vi "ATR.vi"() -> ()   [LabVIEW 2017]
panel:
  out "deleted portion 3":string[](array[string])
  out "ArrEbay 2":string[][](array[string])
  out "output array":string[][](array[string])
  out "ATR 2":string[][](table)=[["Test Communication", "-", "-", "-", "-", ""], ["Set S/N", "-", "-", "-", "-", ""], ["Set Board Number", "-", "-", "-", "-", ""], [" ", "", "", "", "", ""], ["Test Communication", "-", "-", "-", "-", ""], ["Get S/N", "-", "-", "-", "", ""], ["Get Board Number", "-", "-", "-", "", ""], ["Get FW", "-", "-", "-", "", ""], ["Enable Motor", "", "", "", "", ""], ["Small position command", "", "", "", "", ""], ["Measure delta", "", "", "", "", ""], ["Velocity command", "", "", "", "", ""]] caption="ATR"
  out "ATR":string[][](table)=[["Test Communication", "-", "-", "-", "-", ""], ["Set S/N", "-", "-", "-", "-", ""], ["Set Board Number", "-", "-", "-", "-", ""], [" ", "", "", "", "", ""], ["Test Communication", "-", "-", "-", "-", ""], ["Get S/N", "-", "-", "-", "", ""], ["Get Board Number", "-", "-", "-", "", ""], ["Get FW", "-", "-", "-", "", ""], ["Enable Motor", "", "", "", "", ""], ["Small position command", "", "", "", "", ""], ["Measure delta", "", "", "", "", ""], ["Velocity command", "", "", "", "", ""]]
  out "Array 2":string[](array[string])
  out "Array":string[](array[string])
  out "deleted portion 2":string[](array[string])
  out "deleted portion":string[](array[string])
  out "ArrAHU":string[][](array[string])
  out "ArrEbay":string[][](array[string])
  out "Mort Temp":string[][](array[string])
  out "Aux":string[][](array[string])
  out "Burnin":string[][](array[string])
  out "Temp Algo":string[][](array[string])
  out "Speed":string[][](array[string])
  out "Tempreature calibration":string[][](array[string])
  out "StopTime":string[][](array[string])
  out "Enable":string[][](array[string])
  out "Communication":string[][](array[string])
  out "Visual Inspection":string[][](array[string])
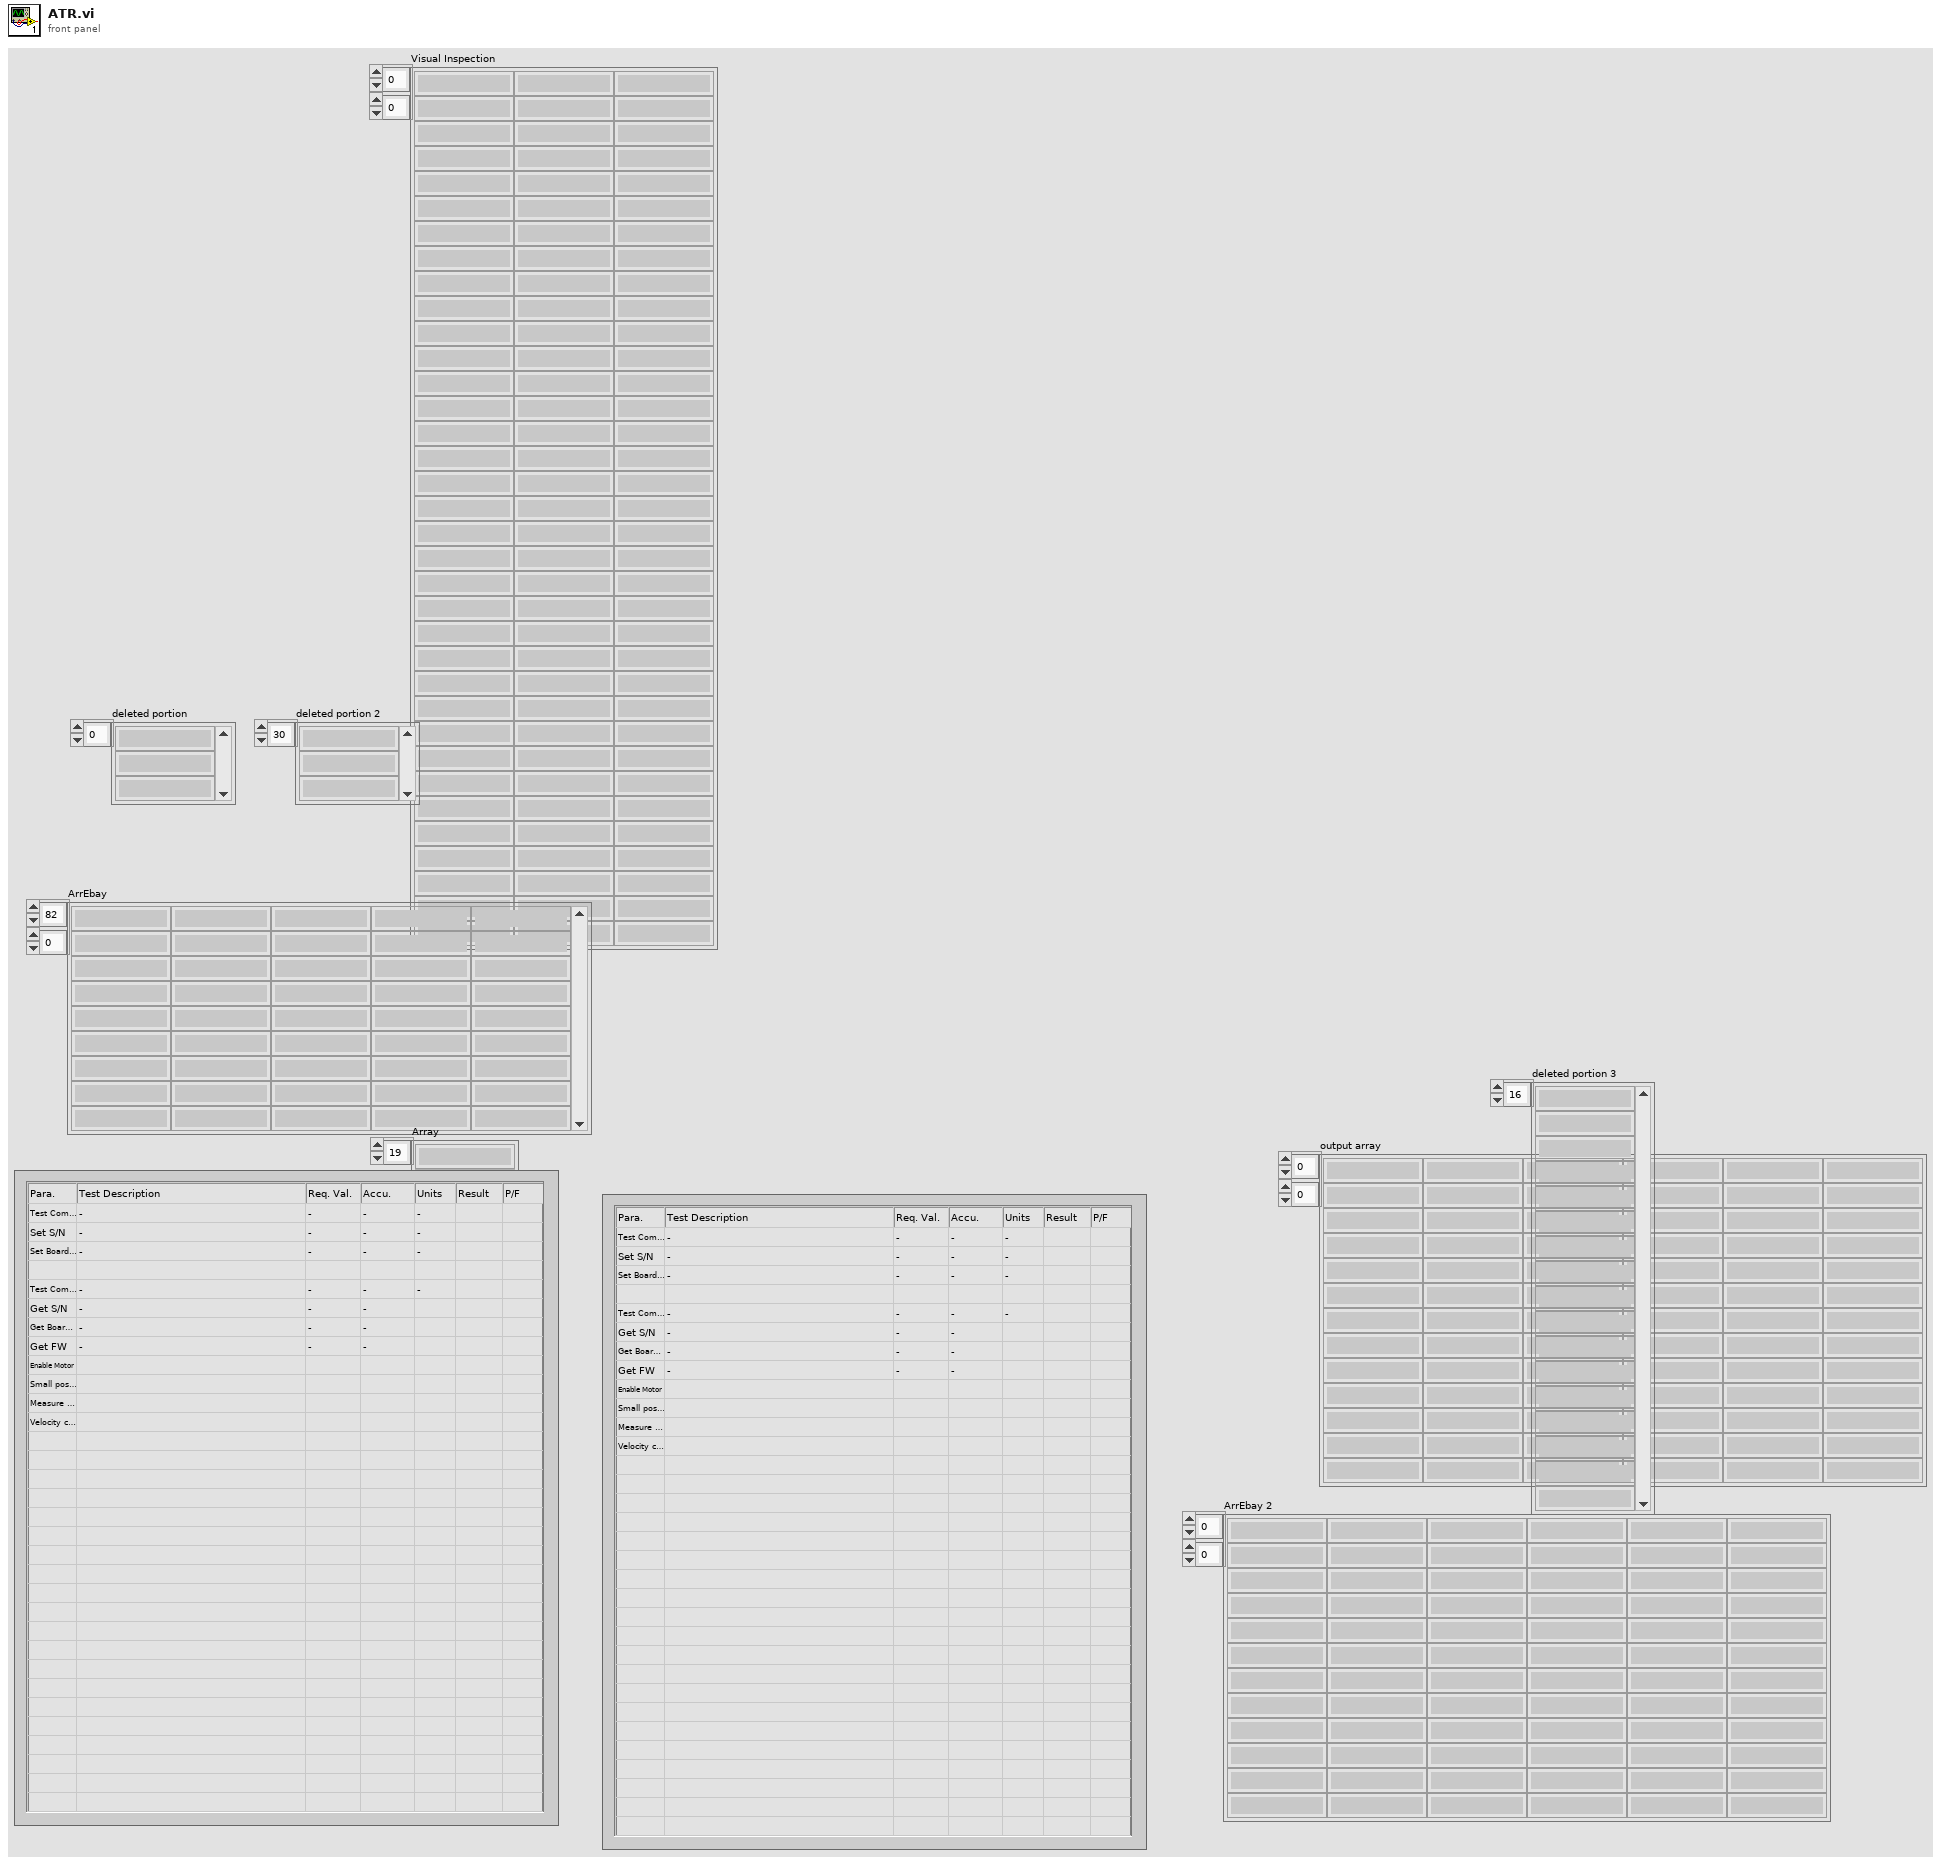
[diagram p1: front panel]
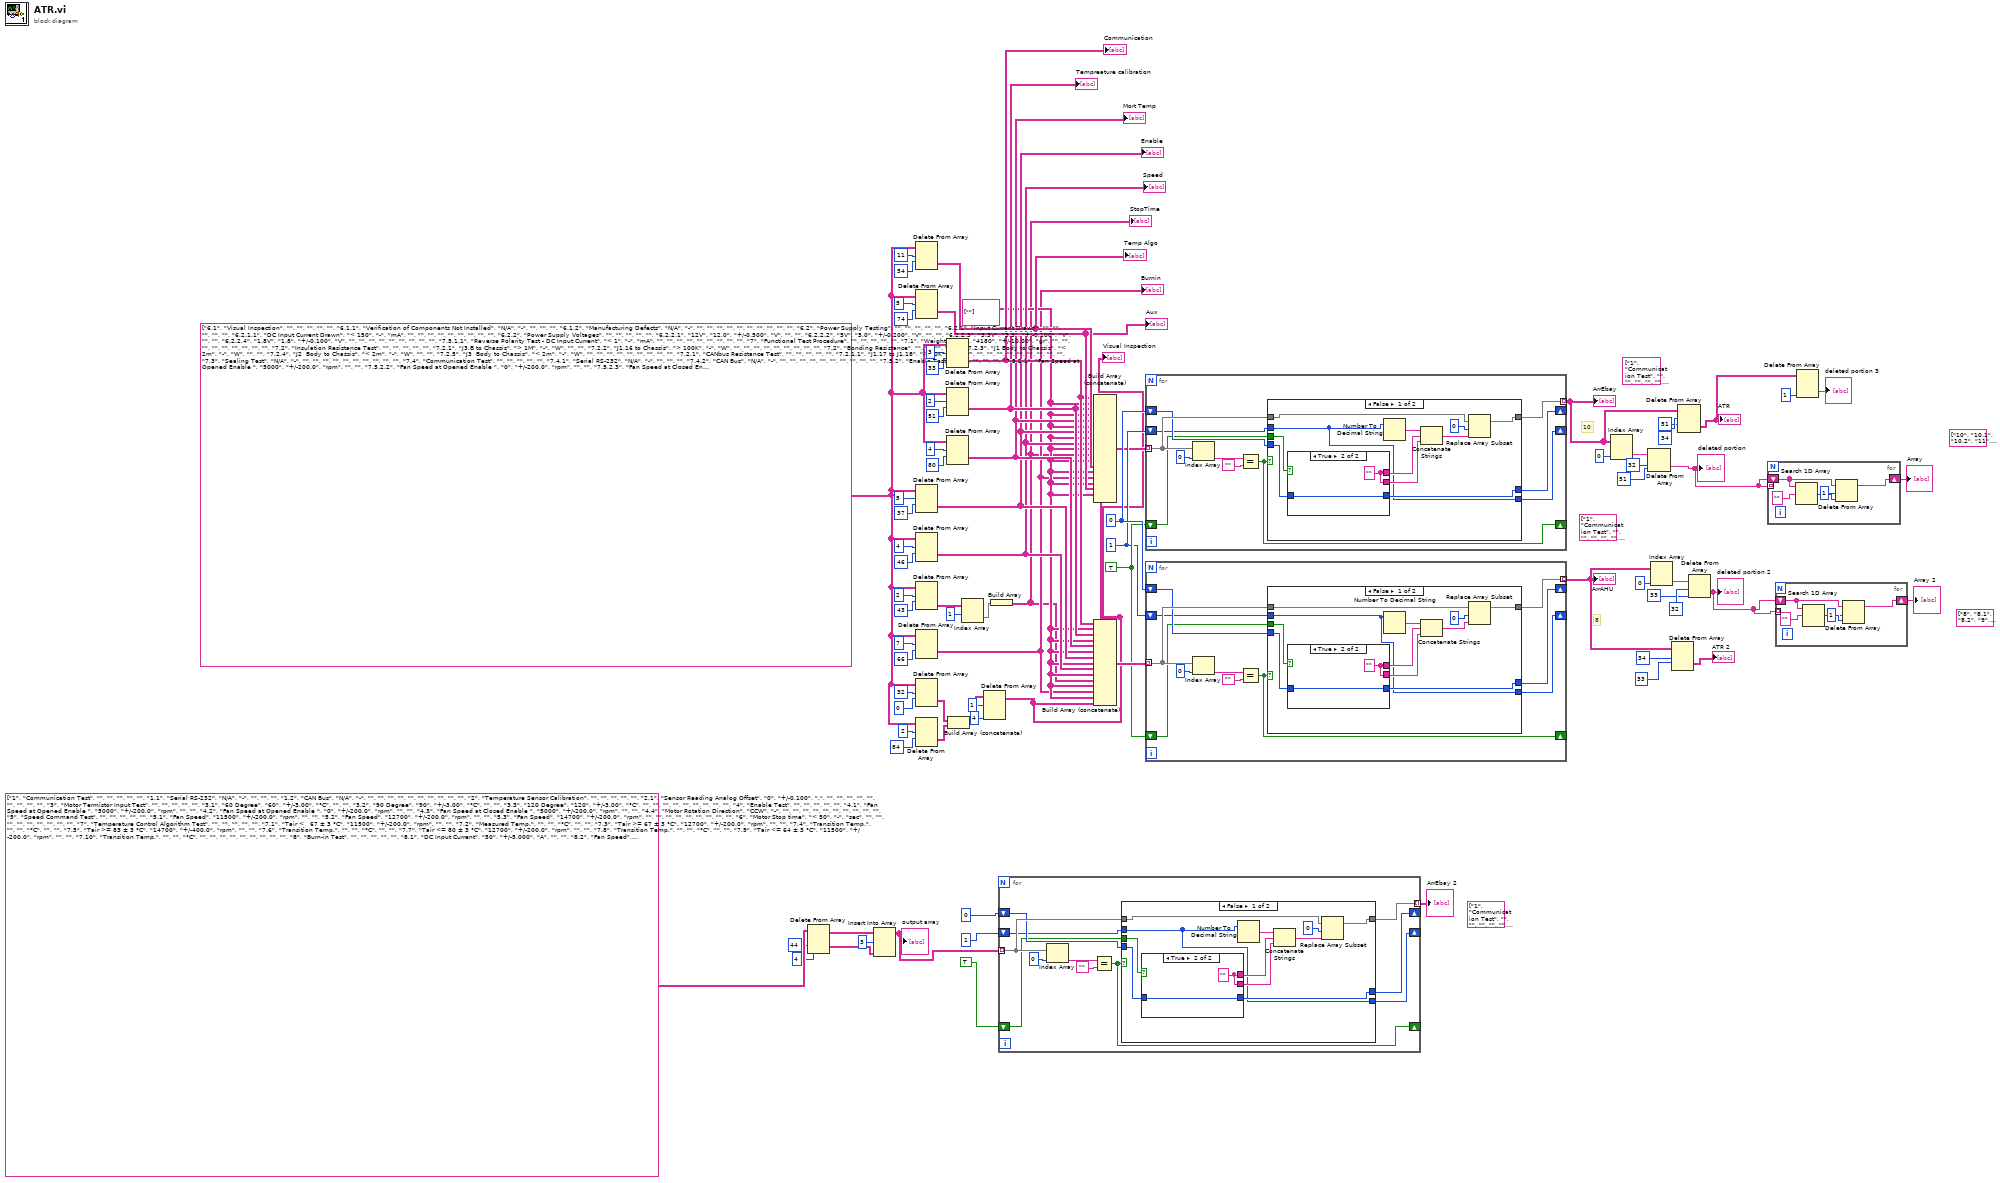
[diagram p0: block diagram]
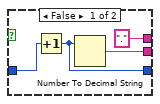
[diagram p2: hidden frame]
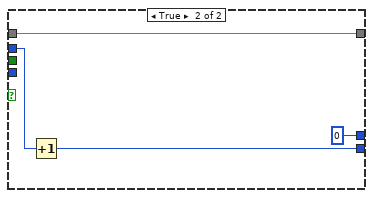
[diagram p3: hidden frame]
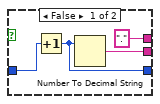
[diagram p4: hidden frame]
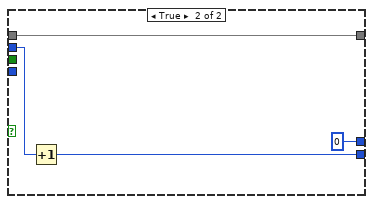
[diagram p5: hidden frame]
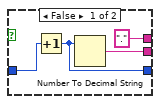
[diagram p6: hidden frame]
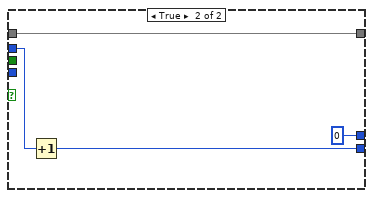
[diagram p7: hidden frame]
diagram:
  (unwired) string[][] [["1", "Communication Test", "", "", "", "", ""], ["1.1", "Serial RS-232", "N/A", "-", "", "", ""], ["1.2", "CAN Bus", "N/A", "-", "", "", ""], ["", "", "", "", "", "", ""], ["2", "Auxiliary Fan Test", "", "", "", "", ""], ["2.1", "Fan status-ON", "ON", "-", "-", "", ""], ["2.2", "Fan status-OFF", "OFF", "-", "-", "", ""], ["", "", "", "", "", "", ""], ["3", "Temperature Sensor Calibration", "", "", "", "", ""], ["3.1", "Sensor Reading Analog Offset", "0", "+/-0.100", ".", "", ""], ["", "", "", "", "", "", ""], ["4", "Motor Termistor Input Test", "", "", "", "", ""], ["4.1", "60 Degree", "60", "+/-3.00", "°C", "", ""], ["4.2", "90 Degree", "90", "+/-3.00", "°C", "", ""], ["4.3", "120 Degree", "120", "+/-3.00", "°C", "", ""], ["", "", "", "", "", "", ""], ["5", "Enable Test", "", "", "", "", ""], ["5.1", "Fan Speed at Opened Enable ", "5000", "+/-200.0", "rpm", "", ""], ["5.2", "Fan Speed at Opened Enable ", "0", "+/-200.0", "rpm", "", ""], ["5.3", "Fan Speed at Closed Enable ", "5000", "+/-200.0", "rpm", "", ""], ["5.4", "Motor Rotation Direction", "CCW", "-", "", "", ""], ["", "", "", "", "", "", ""], ["6", "Speed Command Test", "", "", "", "", ""], ["6.1", "Fan Speed", "11500", "+/-200.0", "rpm", "", ""], ["6.2", "Fan Speed", "12700", "+/-200.0", "rpm", "", ""], ["6.3", "Fan Speed", "14700", "+/-200.0", "rpm", "", ""], ["", "", "", "", "", "", ""], ["7", "Motor Stop time", "< 50", "-", "sec", "", ""], ["", "", "", "", "", "", ""], ["8", "Temperature Control Algorithm Test", "", "", "", "", ""], ["8.1", "Tair <   67 ± 3 °C", "11500", "+/-200.0", "rpm", "", ""], ["8.2", "Measured Temp.", "", "", "°C", "", ""], ["8.3", "Tair >= 67 ± 3 °C", "12700", "+/-200.0", "rpm", "", ""], ["8.4", "Transition Temp.", "", "", "°C", "", ""], ["8.5", "Tair >= 83 ± 3 °C", "14700", "+/-400.0", "rpm", "", ""], ["8.6", "Transition Temp.", "", "", "°C", "", ""], ["8.7", "Tair <= 80 ± 3 °C", "12700", "+/-200.0", "rpm", "", ""], ["8.8", "Transition Temp.", "", "", "°C", "", ""], ["8.9", "Tair <= 64 ± 3 °C", "11500", "+/-200.0", "rpm", "", ""], ["8.10", "Transition Temp.", "", "", "°C", "", ""], ["", "", "", "", "", "", ""], ["9", "Burn-in Test", "", "", "", "", ""], ["9.1", "DC Input Current", "50", "+/-5.000", "A", "", ""], ["9.2", "Fan Speed", "14700", "+/-200.0", "rpm", "", ""], ["9.3", "Ambient Temperature", "25", "+/-13.00", "°C", "", ""], ["9.4", "After 10 min of operation", "", "-", "°C", "", ""], ["9.5", "After 20 min of operation", "", "-", "°C", "", ""], ["9.6", "After 30 min of operation", "", "-", "°C", "", ""], ["", "", "", "", "", "", ""], ["10", "Visual Inspection", "", "", "", "", ""], ["10.1", "Verification of Components Not Installed", "N/A", "-", "", "", ""], ["10.2", "Manufacturing Defects", "N/A", "-", "", "", ""], ["", "", "", "", "", "", ""], ["11", "Power Supply Testing", "", "", "", "", ""], ["11.1", "DC Input Current Drawn", "150", "+/-10.00", "mA", "", ""], ["", "", "", "", "", "", ""], ["12", "Power Supply Voltages", "", "", "", "", ""], ["12.1", "12V", "12.0", "+/-0.500", "V", "", ""], ["12.2", "5V", "5.0", "+/-0.200", "V", "", ""], ["12.3", "3.3V", "3.3", "+/-0.100", "V", "", ""], ["12.4", "1.8V", "1.8", "+/-0.100", "V", "", ""], ["", "", "", "", "", "", ""], ["13", "Reverse Polarity Test - DC Input Current", "< 1", "-", "mA", "", ""], ["", "", "", "", "", "", ""], ["14", "Functional Test Procedure", "", "", "", "", ""], ["14.1", "Weight Check", "4180", "+/-100.0", "gr", "", ""], ["", "", "", "", "", "", ""], ["15", "Insulation Resistance Test", "", "", "", "", ""], ["15.1", "J3.B to Chassis", "> 1M", "-", "ohms", "", ""], ["15.2", "J1.16 to Chassis", "> 100K", "-", "ohms", "", ""], ["", "", "", "", "", "", ""], ["16", "Bonding Resistance", "", "", "", "", ""], ["16.1", "J1 Body to Chassis", "< 2m", "-", "ohms", "", ""], ["16.2", "J2  Body to Chassis", "< 2m", "-", "ohms", "", ""], ["16.3", "J3  Body to Chassis", "< 2m", "-", "ohms", "", ""], ["", "", "", "", "", "", ""], ["17", "CANbus Resistance Test", "", "", "", "", ""], ["17.1", "J1.17 to J1.18", "> 10K", "-", "ohms", "", ""], ["", "", "", "", "", "", ""], ["18", "Sealing Test", "N/A", "-", "", "", ""], ["", "", "", "", "", "", ""], ["19", "Mounting Holes Test - Jig Fit", "214", "-", "mm", "", ""]] ("ArrEbay 3")
  (unwired) string[] ["8", "8.1", "8.2", "9", "9.1", "9.2", "10", "10.1", "10.2", "10.3", "10.4", "11", "12", "12.1", "13", "13.1", "13.2", "14", "14.1", "14.2", "14.3", "15", "15.1", "16"] ("Array 3")
  (unwired) string[] ["10", "10.1", "10.2", "11", "11.1", "11.2", "12", "12.1", "12.2", "12.3", "12.4", "13", "14", "14.1", "15", "15.1", "15.2", "16", "16.1", "16.2", "16.3", "17", "17.1", "18"] ("Array 4")
  (unwired) string[][] [["1", "Communication Test", "", "", "", "", ""], ["1.1", "Serial RS-232", "N/A", "-", "", "", ""], ["1.2", "CAN Bus", "N/A", "-", "", "", ""], ["", "", "", "", "", "", ""], ["2", "Temperature Sensor Calibration", "", "", "", "", ""], ["2.1", "Sensor Reading Analog Offset", "0", "+/-0.100", ".", "", ""], ["", "", "", "", "", "", ""], ["3", "Motor Termistor Input Test", "", "", "", "", ""], ["3.1", "60 Degree", "60", "+/-3.00", "C", "", ""], ["3.2", "90 Degree", "90", "+/-3.00", "C", "", ""], ["3.3", "120 Degree", "120", "+/-3.00", "C", "", ""], ["", "", "", "", "", "", ""], ["4", "Enable Test", "", "", "", "", ""], ["4.1", "Fan Speed at Opened Enable ", "5000", "+/-200.0", "rpm", "", ""], ["4.2", "Fan Speed at Opened Enable ", "0", "+/-200.0", "rpm", "", ""], ["4.3", "Fan Speed at Closed Enable ", "5000", "+/-200.0", "rpm", "", ""], ["4.4", "Motor Rotation Direction", "Counter-clockwise (Inlet)", "-", "", "", ""], ["", "", "", "", "", "", ""], ["5", "Speed Command Test", "", "", "", "", ""], ["5.1", "Fan Speed", "6000", "+/-200.0", "rpm", "", ""], ["5.2", "Fan Speed", "11500", "+/-200.0", "rpm", "", ""], ["5.3", "Fan Speed", "15100", "+/-200.0", "rpm", "", ""], ["", "", "", "", "", "", ""], ["6", "Motor Stop time", "< 50", "-", "sec", "", ""], ["", "", "", "", "", "", ""], ["7", "Temperature Control Algorithm Test", "", "", "", "", ""], ["7.1", "Tair <   68 ± 2 oC", "6000", "+/-200.0", "rpm", "", ""], ["7.2", "Measured Temp.", "", "", "C", "", ""], ["7.3", "Tair >= 68 ± 2 oC", "11500", "+/-200.0", "rpm", "", ""], ["7.4", "Transition Temp.", "", "", "C", "", ""], ["7.5", "Tair >= 88 ± 2 oC", "15100", "+/-400.0", "rpm", "", ""], ["7.6", "Transition Temp.", "", "", "C", "", ""], ["7.7", "Tair <= 80 ± 2 oC", "11500", "+/-200.0", "rpm", "", ""], ["7.8", "Transition Temp.", "", "", "C", "", ""], ["7.9", "Tair <= 60 ± 2 oC", "6000", "+/-200.0", "rpm", "", ""], ["7.10", "Transition Temp.", "", "", "C", "", ""], ["", "", "", "", "", "", ""], ["8", "Burn-in Test", "", "", "", "", ""], ["8.1", "DC Input Current", "50", "+/-5.000", "A", "", ""], ["8.2", "Fan Speed", "15100", "+/-200.0", "rpm", "", ""], ["8.3", "Ambient Temperature", "25", "+/-13.00", "C", "", ""], ["8.4", "After 10 min of operation", "", "-", "C", "", ""], ["8.5", "After 20 min of operation", "", "-", "C", "", ""], ["8.6", "After 30 min of operation", "", "-", "C", "", ""], ["", "", "", "", "", "", ""], ["9", "Auxiliary Fan Test", "", "", "", "", ""], ["9.1", "Auxiliary Cooling Fan ON", "60", "+/-2.00", "C", "", ""], ["9.2", "Fan status", "ON", "-", "-", "", ""], ["9.3", "Auxiliary Cooling Fan OFF", "55", "+/-2.00", "C", "", ""], ["9.4", "Fan status", "OFF", "-", "-", "", ""], ["", "", "", "", "", "", ""], ["10", "Visual Inspection", "", "", "", "", ""], ["10.1", "Verification of Components Not Installed", "N/A", "-", "", "", ""], ["10.2", "Manufacturing Defects", "N/A", "-", "", "", ""], ["", "", "", "", "", "", ""], ["11", "Power Supply Testing", "", "", "", "", ""], ["11.1", "Input Current Drawn", "", "", "", "", ""], ["11.2", "DC Input Current", "< 150", "-", "mA", "", ""], ["", "", "", "", "", "", ""], ["12", "Power Supply Voltages", "", "", "", "", ""], ["12.1", "12V", "12.0", "+/-0.500", "V", "", ""], ["12.2", "5V", "5.0", "+/-0.200", "V", "", ""], ["12.3", "3.3V", "3.3", "+/-0.100", "V", "", ""], ["12.4", "1.8V", "1.8", "+/-0.100", "V", "", ""], ["", "", "", "", "", "", ""], ["13", "Reverse Polarity Test - DC Input Current", "< 1", "-", "mA", "", ""], ["", "", "", "", "", "", ""], ["14", "Functional Test Procedure", "", "", "", "", ""], ["14.1", "Weight Check", "4180", "+/-10.00", "gr", "", ""], ["", "", "", "", "", "", ""], ["15", "Insulation Resistance Test", "", "", "", "", ""], ["15.1", "J3.B to Chassis", "> 1M", "-", "W", "", ""], ["15.2", "J1.16 to Chassis", "> 100K", "-", "W", "", ""], ["", "", "", "", "", "", ""], ["16", "Bonding Resistance", "", "", "", "", ""], ["16.1", "J1 Body to Chassis", "< 2m", "-", "W", "", ""], ["16.2", "J2  Body to Chassis", "< 2m", "-", "W", "", ""], ["16.3", "J3  Body to Chassis", "< 2m", "-", "W", "", ""], ["", "", "", "", "", "", ""], ["17", "CANbus Resistance Test", "", "", "", "", ""], ["17.1", "J1.17 to J1.18", "> 10K", "-", "W", "", ""], ["", "", "", "", "", "", ""], ["18", "Sealing Test", "N/A", "-", "", "", ""]] ("ArrEbay 2")
  (unwired) string[][] [["1", "Communication Test", "", "", "", "", ""], ["1.1", "Serial RS-232", "N/A", "-", "", "", ""], ["1.2", "CAN Bus", "N/A", "-", "", "", ""], ["", "", "", "", "", "", ""], ["2", "Temperature Sensor Calibration", "", "", "", "", ""], ["2.1", "Sensor Reading Analog Offset", "0", "+/-0.100", ".", "", ""], ["", "", "", "", "", "", ""], ["3", "Motor Termistor Input Test", "", "", "", "", ""], ["3.1", "60 Degree", "60", "+/-3.00", "C", "", ""], ["3.2", "90 Degree", "90", "+/-3.00", "C", "", ""], ["3.3", "120 Degree", "120", "+/-3.00", "C", "", ""], ["", "", "", "", "", "", ""], ["4", "Enable Test", "", "", "", "", ""], ["4.1", "Fan Speed at Opened Enable ", "5000", "+/-200.0", "rpm", "", ""], ["4.2", "Fan Speed at Opened Enable ", "0", "+/-200.0", "rpm", "", ""], ["4.3", "Fan Speed at Closed Enable ", "5000", "+/-200.0", "rpm", "", ""], ["4.4", "Motor Rotation Direction", "Counter-clockwise (Inlet)", "-", "", "", ""], ["", "", "", "", "", "", ""], ["5", "Speed Command Test", "", "", "", "", ""], ["5.1", "Fan Speed", "6000", "+/-200.0", "rpm", "", ""], ["5.2", "Fan Speed", "11500", "+/-200.0", "rpm", "", ""], ["5.3", "Fan Speed", "15100", "+/-200.0", "rpm", "", ""], ["", "", "", "", "", "", ""], ["6", "Motor Stop time", "< 50", "-", "sec", "", ""], ["", "", "", "", "", "", ""], ["7", "Burn-in Test", "", "", "", "", ""], ["7.1", "DC Input Current", "50", "+/-5.000", "A", "", ""], ["7.2", "Fan Speed", "15100", "+/-200.0", "rpm", "", ""], ["7.3", "Ambient Temperature", "25", "+/-13.00", "C", "", ""], ["7.4", "After 10 min of operation", "", "-", "C", "", ""], ["7.5", "After 20 min of operation", "", "-", "C", "", ""], ["7.6", "After 30 min of operation", "", "-", "C", "", ""], ["", "", "", "", "", "", ""], ["8", "Visual Inspection", "", "", "", "", ""], ["8.1", "Verification of Components Not Installed", "N/A", "-", "", "", ""], ["8.2", "Manufacturing Defects", "N/A", "-", "", "", ""], ["", "", "", "", "", "", ""], ["9", "Power Supply Testing", "", "", "", "", ""], ["9.1", "Input Current Drawn", "", "", "", "", ""], ["9.2", "DC Input Current", "< 150", "-", "mA", "", ""], ["", "", "", "", "", "", ""], ["10", "Power Supply Voltages", "", "", "", "", ""], ["10.1", "12V", "12.0", "+/-0.500", "V", "", ""], ["10.2", "5V", "5.0", "+/-0.200", "V", "", ""], ["10.3", "3.3V", "3.3", "+/-0.100", "V", "", ""], ["10.4", "1.8V", "1.8", "+/-0.100", "V", "", ""], ["", "", "", "", "", "", ""], ["11", "Reverse Polarity Test - DC Input Current", "< 1", "-", "mA", "", ""], ["", "", "", "", "", "", ""], ["12", "Functional Test Procedure", "", "", "", "", ""], ["12.1", "Weight Check", "4180", "+/-10.00", "gr", "", ""], ["", "", "", "", "", "", ""], ["13", "Insulation Resistance Test", "", "", "", "", ""], ["13.1", "J3.B to Chassis", "> 1M", "-", "W", "", ""], ["13.2", "J1.16 to Chassis", "> 100K", "-", "W", "", ""], ["", "", "", "", "", "", ""], ["14", "Bonding Resistance", "", "", "", "", ""], ["14.1", "J1 Body to Chassis", "< 2m", "-", "W", "", ""], ["14.2", "J2  Body to Chassis", "< 2m", "-", "W", "", ""], ["14.3", "J3  Body to Chassis", "< 2m", "-", "W", "", ""], ["", "", "", "", "", "", ""], ["15", "CANbus Resistance Test", "", "", "", "", ""], ["15.1", "J1.17 to J1.18", "> 10K", "-", "W", "", ""], ["", "", "", "", "", "", ""], ["16", "Sealing Test", "N/A", "-", "", "", ""]] ("ArrAHU 2")
  w53 = string[][] [[""]] ("array")
  w50 = TRUE
  w49 = 1
  w51 = 0
  w21 = string[][] [["6.1", "Visual Inspection", "", "", "", "", ""], ["6.1.1", "Verification of Components Not Installed", "N/A", "-", "", "", ""], ["6.1.2", "Manufacturing Defects", "N/A", "-", "", "", ""], ["", "", "", "", "", "", ""], ["6.2", "Power Supply Testing", "", "", "", "", ""], ["6.2.1", "Input Current Drawn", "", "", "", "", ""], ["6.2.1.1", "DC Input Current Drawn", "< 150", "-", "mA", "", ""], ["", "", "", "", "", "", ""], ["6.2.2", "Power Supply Voltages", "", "", "", "", ""], ["6.2.2.1", "12V", "12.0", "+/-0.500", "V", "", ""], ["6.2.2.2", "5V", "5.0", "+/-0.200", "V", "", ""], ["6.2.2.3", "3.3V", "3.3", "+/-0.100", "V", "", ""], ["6.2.2.4", "1.8V", "1.8", "+/-0.100", "V", "", ""], ["", "", "", "", "", "", ""], ["7.5.1.1", "Reverse Polarity Test - DC Input Current", "< 1", "-", "mA", "", ""], ["", "", "", "", "", "", ""], ["7", "Functional Test Procedure", "", "", "", "", ""], ["7.1", "Weight Check", "4180", "+/-10.00", "gr", "", ""], ["", "", "", "", "", "", ""], ["7.2", "Insulation Resistance Test", "", "", "", "", ""], ["7.2.1", "J3.B to Chassis", "> 1M", "-", "W", "", ""], ["7.2.2", "J1.16 to Chassis", "> 100K", "-", "W", "", ""], ["", "", "", "", "", "", ""], ["7.2", "Bonding Resistance", "", "", "", "", ""], ["7.2.3", "J1 Body to Chassis", "< 2m", "-", "W", "", ""], ["7.2.4", "J2  Body to Chassis", "< 2m", "-", "W", "", ""], ["7.2.5", "J3  Body to Chassis", "< 2m", "-", "W", "", ""], ["", "", "", "", "", "", ""], ["7.2.1", "CANbus Resistance Test", "", "", "", "", ""], ["7.2.1.1", "J1.17 to J1.18", "> 10K", "-", "W", "", ""], ["", "", "", "", "", "", ""], ["7.3", "Sealing Test", "N/A", "-", "", "", ""], ["", "", "", "", "", "", ""], ["7.4", "Communication Test", "", "", "", "", ""], ["7.4.1", "Serial RS-232", "N/A", "-", "", "", ""], ["7.4.2", "CAN Bus", "N/A", "-", "", "", ""], ["", "", "", "", "", "", ""], ["7.5.2", "Enable Test", "", "", "", "", ""], ["7.5.2.1", "Fan Speed at Opened Enable ", "5000", "+/-200.0", "rpm", "", ""], ["7.5.2.2", "Fan Speed at Opened Enable ", "0", "+/-200.0", "rpm", "", ""], ["7.5.2.3", "Fan Speed at Closed Enable ", "5000", "+/-200.0", "rpm", "", ""], ["7.5.2.4", "Motor Rotation Direction", "Counter-clockwise (Inlet)", "-", "", "", ""], ["", "", "", "", "", "", ""], ["7.5.3", "Stop Time Test ", "", "", "", "", ""], ["7.5.3.1", "Motor Stop time", "< 50", "-", "sec", "", ""], ["", "", "", "", "", "", ""], ["7.5.4", "Speed Command Test", "", "", "", "", ""], ["7.5.4.1", "Fan Speed", "6000", "+/-200.0", "rpm", "", ""], ["7.5.4.2", "Fan Speed", "11500", "+/-200.0", "rpm", "", ""], ["7.5.4.3", "Fan Speed", "15100", "+/-200.0", "rpm", "", ""], ["", "", "", "", "", "", ""], ["7.5.5", "Temperature Sensor Calibration", "", "", "", "", ""], ["7.5.5.1", "Sensor Reading Analog Offset", "0", "+/-0.100", ".", "", ""], ["", "", "", "", "", "", ""], ["7.5.6", "Temperature Control Algorithm Test", "", "", "", "", ""], ["7.5.6.1", "Tair <   68 ± 2 oC", "6000", "+/-200.0", "rpm", "", ""], ["7.5.6.2", "Measured Temp.", "", "", "C", "", ""], ["7.5.6.3", "Tair >= 68 ± 2 oC", "11500", "+/-200.0", "rpm", "", ""], ["7.5.6.4", "Transition Temp.", "", "", "C", "", ""], ["7.5.6.5", "Tair >= 88 ± 2 oC", "15100", "+/-400.0", "rpm", "", ""], ["7.5.6.6", "Transition Temp.", "", "", "C", "", ""], ["7.5.6.7", "Tair <= 80 ± 2 oC", "11500", "+/-200.0", "rpm", "", ""], ["7.5.6.8", "Transition Temp.", "", "", "C", "", ""], ["7.5.6.9", "Tair <= 60 ± 2 oC", "6000", "+/-200.0", "rpm", "", ""], ["7.5.6.10", "Transition Temp.", "", "", "C", "", ""], ["", "", "", "", "", "", ""], ["7.5.7", "Burn-in Test", "", "", "", "", ""], ["7.5.7.1", "DC Input Current", "50", "+/-5.000", "A", "", ""], ["7.5.7.2", "Fan Speed", "15100", "+/-200.0", "rpm", "", ""], ["7.5.7.3", "Ambient Temperature", "25", "+/-13.00", "C", "", ""], ["7.5.7.4", "After 10 min of operation", "", "-", "C", "", ""], ["7.5.7.5", "After 20 min of operation", "", "-", "C", "", ""], ["7.5.7.6", "After 30 min of operation", "", "-", "C", "", ""], ["", "", "", "", "", "", ""], ["8", "Auxiliary Fan Test", "", "", "", "", ""], ["8.1", "Auxiliary Cooling Fan ON", "60", "+/-2.00", "C", "", ""], ["8.2", "Fan status", "ON", "-", "-", "", ""], ["8.3", "Auxiliary Cooling Fan OFF", "55", "+/-2.00", "C", "", ""], ["8.4", "Fan status", "OFF", "-", "-", "", ""], ["", "", "", "", "", "", ""], ["9", "Motor Termistor Input Test", "", "", "", "", ""], ["9.1", "60 Degree", "60", "+/-3.00", "C", "", ""], ["9.2", "90 Degree", "90", "+/-3.00", "C", "", ""], ["9.3", "120 Degree", "120", "+/-3.00", "C", "", ""], ["", "", "", "", "", "", ""], ["10", "Mounting Holes Test - Jig Fit", "214", "-", "mm", "", ""]] ("data")
  # "8"
  # "10"
  n1 = Delete From Array(array=string[][] [["1", "Communication Test", "", "", "", "", ""], ["1.1", "Serial RS-232", "N/A", "-", "", "", ""], ["1.2", "CAN Bus", "N/A", "-", "", "", ""], ["", "", "", "", "", "", ""], ["2", "Temperature Sensor Calibration", "", "", "", "", ""], ["2.1", "Sensor Reading Analog Offset", "0", "+/-0.100", ".", "", ""], ["", "", "", "", "", "", ""], ["3", "Motor Termistor Input Test", "", "", "", "", ""], ["3.1", "60 Degree", "60", "+/-3.00", "°C", "", ""], ["3.2", "90 Degree", "90", "+/-3.00", "°C", "", ""], ["3.3", "120 Degree", "120", "+/-3.00", "°C", "", ""], ["", "", "", "", "", "", ""], ["4", "Enable Test", "", "", "", "", ""], ["4.1", "Fan Speed at Opened Enable ", "5000", "+/-200.0", "rpm", "", ""], ["4.2", "Fan Speed at Opened Enable ", "0", "+/-200.0", "rpm", "", ""], ["4.3", "Fan Speed at Closed Enable ", "5000", "+/-200.0", "rpm", "", ""], ["4.4", "Motor Rotation Direction", "CCW", "-", "", "", ""], ["", "", "", "", "", "", ""], ["5", "Speed Command Test", "", "", "", "", ""], ["5.1", "Fan Speed", "11500", "+/-200.0", "rpm", "", ""], ["5.2", "Fan Speed", "12700", "+/-200.0", "rpm", "", ""], ["5.3", "Fan Speed", "14700", "+/-200.0", "rpm", "", ""], ["", "", "", "", "", "", ""], ["6", "Motor Stop time", "< 50", "-", "sec", "", ""], ["", "", "", "", "", "", ""], ["7", "Temperature Control Algorithm Test", "", "", "", "", ""], ["7.1", "Tair <   67 ± 3 °C", "11500", "+/-200.0", "rpm", "", ""], ["7.2", "Measured Temp.", "", "", "°C", "", ""], ["7.3", "Tair >= 67 ± 3 °C", "12700", "+/-200.0", "rpm", "", ""], ["7.4", "Transition Temp.", "", "", "°C", "", ""], ["7.5", "Tair >= 83 ± 3 °C", "14700", "+/-400.0", "rpm", "", ""], ["7.6", "Transition Temp.", "", "", "°C", "", ""], ["7.7", "Tair <= 80 ± 3 °C", "12700", "+/-200.0", "rpm", "", ""], ["7.8", "Transition Temp.", "", "", "°C", "", ""], ["7.9", "Tair <= 64 ± 3 °C", "11500", "+/-200.0", "rpm", "", ""], ["7.10", "Transition Temp.", "", "", "°C", "", ""], ["", "", "", "", "", "", ""], ["8", "Burn-in Test", "", "", "", "", ""], ["8.1", "DC Input Current", "50", "+/-5.000", "A", "", ""], ["8.2", "Fan Speed", "14700", "+/-200.0", "rpm", "", ""], ["8.3", "Ambient Temperature", "25", "+/-13.00", "°C", "", ""], ["8.4", "After 10 min of operation", "", "-", "°C", "", ""], ["8.5", "After 20 min of operation", "", "-", "°C", "", ""], ["8.6", "After 30 min of operation", "", "-", "°C", "", ""], ["", "", "", "", "", "", ""], ["9", "Auxiliary Fan Test", "", "", "", "", ""], ["9.1", "Fan status-ON", "ON", "-", "-", "", ""], ["9.2", "Fan status-OFF", "OFF", "-", "-", "", ""], ["", "", "", "", "", "", ""], ["10", "Visual Inspection", "", "", "", "", ""], ["10.1", "Verification of Components Not Installed", "N/A", "-", "", "", ""], ["10.2", "Manufacturing Defects", "N/A", "-", "", "", ""], ["", "", "", "", "", "", ""], ["11", "Power Supply Testing", "", "", "", "", ""], ["11.1", "DC Input Current Drawn", "150", "+/-10.00", "mA", "", ""], ["", "", "", "", "", "", ""], ["12", "Power Supply Voltages", "", "", "", "", ""], ["12.1", "12V", "12.0", "+/-0.500", "V", "", ""], ["12.2", "5V", "5.0", "+/-0.200", "V", "", ""], ["12.3", "3.3V", "3.3", "+/-0.100", "V", "", ""], ["12.4", "1.8V", "1.8", "+/-0.100", "V", "", ""], ["", "", "", "", "", "", ""], ["13", "Reverse Polarity Test - DC Input Current", "< 1", "-", "mA", "", ""], ["", "", "", "", "", "", ""], ["14", "Functional Test Procedure", "", "", "", "", ""], ["14.1", "Weight Check", "4180", "+/-100.0", "gr", "", ""], ["", "", "", "", "", "", ""], ["15", "Insulation Resistance Test", "", "", "", "", ""], ["15.1", "J3.B to Chassis", "> 1M", "-", "ohms", "", ""], ["15.2", "J1.16 to Chassis", "> 100K", "-", "ohms", "", ""], ["", "", "", "", "", "", ""], ["16", "Bonding Resistance", "", "", "", "", ""], ["16.1", "J1 Body to Chassis", "< 2m", "-", "ohms", "", ""], ["16.2", "J2  Body to Chassis", "< 2m", "-", "ohms", "", ""], ["16.3", "J3  Body to Chassis", "< 2m", "-", "ohms", "", ""], ["", "", "", "", "", "", ""], ["17", "CANbus Resistance Test", "", "", "", "", ""], ["17.1", "J1.17 to J1.18", "> 10K", "-", "ohms", "", ""], ["", "", "", "", "", "", ""], ["18", "Sealing Test", "N/A", "-", "", "", ""], ["", "", "", "", "", "", ""], ["19", "Mounting Holes Test - Jig Fit", "214", "-", "mm", "", ""]] ("ArrEbay 2"), length=4, index (row)=44) -> (deleted portion=w10:string[][], array with subset deleted=w11:string[][])  [unwired: 1 in]
  n2 = Insert Into Array(array=w11, index (row)=3, new element=w10) -> (w8:string[][])  [unwired: 1 in]
  "output array" <- w8
  n3 = Delete From Array(array=w21, length=11, index (row)=54) -> (deleted portion=w60:string[][])  [unwired: 1 in, 1 out]
  "Temp Algo" <- w60
  n4 = Delete From Array(array=w21, length=5, index (row)=74) -> (deleted portion=w59:string[][])  [unwired: 1 in, 1 out]
  "Aux" <- w59
  n5 = Delete From Array(array=w21, length=5, index (row)=37) -> (deleted portion=w55:string[][])  [unwired: 1 in, 1 out]
  "Enable" <- w55
  n6 = Delete From Array(array=w21, length=4, index (row)=46) -> (deleted portion=w54:string[][])  [unwired: 1 in, 1 out]
  "Speed" <- w54
  n7 = Delete From Array(array=w21, length=2, index (row)=43) -> (deleted portion=w46:string[][])  [unwired: 1 in, 1 out]
  n8 = Delete From Array(array=w21, length=7, index (row)=66) -> (deleted portion=w47:string[][])  [unwired: 1 in, 1 out]
  "Burnin" <- w47
  n9 = Delete From Array(array=w21, length=32, index (row)=0) -> (deleted portion=w20:string[][])  [unwired: 1 in, 1 out]
  n10 = Delete From Array(array=w21, length=2, index (row)=84) -> (deleted portion=w19:string[][])  [unwired: 1 in, 1 out]
  n11 = Delete From Array(array=w21, length=3, index (row)=33) -> (deleted portion=w58:string[][])  [unwired: 1 in, 1 out]
  "Communication" <- w58
  n12 = Delete From Array(array=w21, length=2, index (row)=51) -> (deleted portion=w57:string[][])  [unwired: 1 in, 1 out]
  "Tempreature calibration" <- w57
  n13 = Delete From Array(array=w21, length=4, index (row)=80) -> (deleted portion=w56:string[][])  [unwired: 1 in, 1 out]
  "Mort Temp" <- w56
  n14 = Build Array (concatenate)(w20, w19) -> (w18:string[][])
  n15 = Index Array(array=w46, index (row)=1) -> (element=w44:string[])  [unwired: 1 in]
  n16 = Delete From Array(array=w18, length=1, index (row)=4) -> (array with subset deleted=w15:string[][])  [unwired: 1 in, 1 out]
  "Visual Inspection" <- w15
  n17 = Build Array(w44) -> (w43:string[][])
  "StopTime" <- w43
  n18 = for {
    tunnel: w8 -> [w90] mode=indexing
    tunnel: [w91] -> w4 mode=indexing
    shift-right: [w85] -> _
    shift-left: 0 -> [w86]
    shift-right: [w83] -> _
    shift-left: 1 -> [w84]
    shift-right: [w82] -> _
    shift-left: TRUE -> [w81]
    n19 = Index Array(array=w90, index=0) -> (element=w88:string)
    n20 = Equal?(x=w88, y="") -> (x = y?=w82:bool)
    n21 = case shown="False" w82 {
      tunnel: w86 -> [w96 _]
      tunnel: [w99 w112] -> w91
      tunnel: w90 -> [w98 w112]
      tunnel: [w97 0] -> w85
      tunnel: w84 -> [w93 w111]
      tunnel: [w93 w110] -> w83
      tunnel: w81 -> [w92 _]
      frame False {
        n22 = case shown="True" w92 {
          tunnel: [w106 w108] -> w101
          tunnel: [w105 w107] -> w97
          tunnel: w96 -> [w104 w107]
          tunnel: ["." ("string") w108] -> w94
          frame False {
            n23 = Increment(x=w104) -> (x+1=w105:i32)
            n24 = Number To Decimal String(number=w105) -> (decimal integer string=w106:string)  [unwired: 1 in]
          }
          frame True {
            w108 = "" ("string")
          }
        }
        n25 = Number To Decimal String(number=w93) -> (decimal integer string=w95:string)  [unwired: 1 in]
        n26 = Concatenate Strings(w95, w94, w101) -> (w100:string)
        n27 = Replace Array Subset(array=w98, new element=w100, index=0) -> (w99:string[])
      }
      frame True {
        n28 = Increment(x=w111) -> (x+1=w110:i32)
      }
    }
  }
  "ArrEbay 2" <- w4
  n29 = Build Array (concatenate)(w58, w53, w57, w53, w56, w53, w55, w53, w54, w53, w43, w53, w60, w53, w47, w53, w59, w53, w15) -> (w48:string[][])
  n30 = Build Array (concatenate)(w58, w53, w57, w53, w56, w53, w55, w53, w54, w53, w43, w53, w47, w53, w15) -> (w52:string[][])
  n31 = for {
    tunnel: w48 -> [w122] mode=indexing
    tunnel: [w123] -> w28 mode=indexing
    shift-right: [w117] -> _
    shift-left: w51 -> [w118]
    shift-right: [w115] -> _
    shift-left: w49 -> [w116]
    shift-right: [w114] -> _
    shift-left: w50 -> [w113]
    n32 = Index Array(array=w122, index=0) -> (element=w120:string)
    n33 = Equal?(x=w120, y="") -> (x = y?=w114:bool)
    n34 = case shown="False" w114 {
      tunnel: w118 -> [w128 _]
      tunnel: [w131 w144] -> w123
      tunnel: w122 -> [w130 w144]
      tunnel: [w129 0] -> w117
      tunnel: w116 -> [w125 w143]
      tunnel: [w125 w142] -> w115
      tunnel: w113 -> [w124 _]
      frame False {
        n35 = case shown="True" w124 {
          tunnel: [w138 w140] -> w133
          tunnel: [w137 w139] -> w129
          tunnel: w128 -> [w136 w139]
          tunnel: ["." ("string") w140] -> w126
          frame False {
            n36 = Increment(x=w136) -> (x+1=w137:i32)
            n37 = Number To Decimal String(number=w137) -> (decimal integer string=w138:string)  [unwired: 1 in]
          }
          frame True {
            w140 = "" ("string")
          }
        }
        n38 = Number To Decimal String(number=w125) -> (decimal integer string=w127:string)  [unwired: 1 in]
        n39 = Concatenate Strings(w127, w126, w133) -> (w132:string)
        n40 = Replace Array Subset(array=w130, new element=w132, index=0) -> (w131:string[])
      }
      frame True {
        n41 = Increment(x=w143) -> (x+1=w142:i32)
      }
    }
  }
  "ArrEbay" <- w28
  n42 = for {
    tunnel: w52 -> [w154] mode=indexing
    tunnel: [w155] -> w24 mode=indexing
    shift-right: [w149] -> _
    shift-left: w51 -> [w150]
    shift-right: [w147] -> _
    shift-left: w49 -> [w148]
    shift-right: [w146] -> _
    shift-left: w50 -> [w145]
    n43 = Index Array(array=w154, index=0) -> (element=w152:string)
    n44 = Equal?(x=w152, y="") -> (x = y?=w146:bool)
    n45 = case shown="False" w146 {
      tunnel: w150 -> [w160 _]
      tunnel: [w163 w176] -> w155
      tunnel: w154 -> [w162 w176]
      tunnel: [w161 0] -> w149
      tunnel: w148 -> [w157 w175]
      tunnel: [w157 w174] -> w147
      tunnel: w145 -> [w156 _]
      frame False {
        n46 = case shown="True" w156 {
          tunnel: [w170 w172] -> w165
          tunnel: [w169 w171] -> w161
          tunnel: w160 -> [w168 w171]
          tunnel: ["." ("string") w172] -> w158
          frame False {
            n47 = Increment(x=w168) -> (x+1=w169:i32)
            n48 = Number To Decimal String(number=w169) -> (decimal integer string=w170:string)  [unwired: 1 in]
          }
          frame True {
            w172 = "" ("string")
          }
        }
        n49 = Number To Decimal String(number=w157) -> (decimal integer string=w159:string)  [unwired: 1 in]
        n50 = Concatenate Strings(w159, w158, w165) -> (w164:string)
        n51 = Replace Array Subset(array=w162, new element=w164, index=0) -> (w163:string[])
      }
      frame True {
        n52 = Increment(x=w175) -> (x+1=w174:i32)
      }
    }
  }
  "ArrAHU" <- w24
  n53 = Index Array(array=w28, index (col)=0 ("disabled index (col)")) -> (element=w41:string[])  [unwired: 1 in]
  n54 = Delete From Array(array=w41, length=32, index=51) -> (deleted portion=w34:string[])  [unwired: 1 out]
  "deleted portion" <- w34
  n55 = Index Array(array=w24, index (col)=0 ("disabled index (col)")) -> (element=w36:string[])  [unwired: 1 in]
  n56 = Delete From Array(array=w24, length=34, index (row)=33 ("index")) -> (deleted portion=→"ATR 2":string[][])  [unwired: 1 in, 1 out]
  n57 = Delete From Array(array=w28, length=34, index (row)=51 ("index")) -> (deleted portion=w3:string[][])  [unwired: 1 in, 1 out]
  "ATR" <- w3
  n58 = Delete From Array(array=w36, length=32, index=33) -> (deleted portion=w31:string[])  [unwired: 1 out]
  "deleted portion 2" <- w31
  n59 = for {
    tunnel: w34 -> [_] mode=indexing
    shift-right: [w177] -> w33
    shift-left: w34 -> [w180]
    n60 = Search 1D Array(1D array=w180, element="") -> (index of element=w179:i32)  [unwired: 1 in]
    n61 = Delete From Array(array=w180, length=1, index=w179) -> (array with subset deleted=w177:string[])  [unwired: 1 out]
  }
  "Array" <- w33
  n62 = for {
    shift-right: [w182] -> w32
    shift-left: w31 -> [w185]
    tunnel: w31 -> [_] mode=indexing
    n63 = Search 1D Array(1D array=w185, element="") -> (index of element=w184:i32)  [unwired: 1 in]
    n64 = Delete From Array(array=w185, length=1, index=w184) -> (array with subset deleted=w182:string[])  [unwired: 1 out]
  }
  "Array 2" <- w32
  n65 = Delete From Array(array=w3, index (col)=1 ("disabled index (col)")) -> (deleted portion=→"deleted portion 3":string[])  [unwired: 2 in, 1 out]
